vi "Parse Response.vi"(8 "error in (no error)":errorcluster, 10 "JSON Request":string, 11 "JSON-RPC in":refnum<class "JSON-RPC.lvclass">) -> (0 "error out":errorcluster, 1 "ids":string[](array[string]), 2 "Results":variant[](array[variant]), 3 "JSON-RPC out":refnum<class "JSON-RPC.lvclass">)   [LabVIEW 2016, in "JSON-RPC.lvclass"]
uses:
  JSON-RPC.lvclass
  JSON-RPC.lvclass/JSON-RPC.ctl
  Request/Request.lvclass
  <vilib>/addons/_JKI.lib/Serialization/JSON/JKI JSON Serialization.lvlib
  <vilib>/Utility/Data Type/NI_Data Type.lvlib
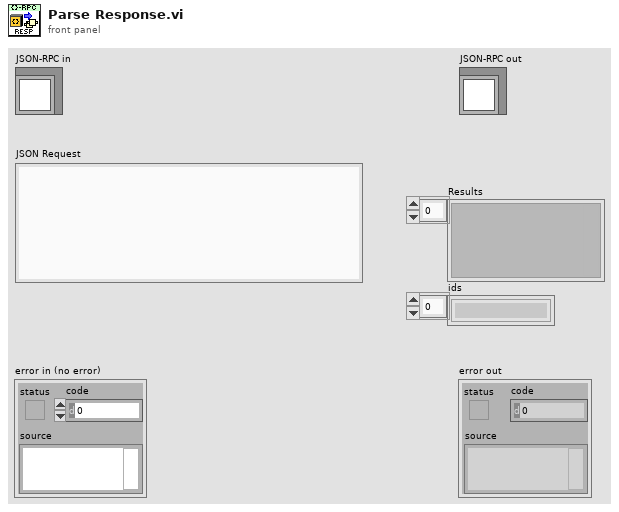
[diagram p1: front panel]
types:
  T1 = typedef "NI_Data Type.lvlib/Data Type.ctl" = enum8{"Invalid Type", "Void", "I8", "I16", "I32", "I64", "U8", "U16", "U32", "U64", "Single Float", "Double Float", "Extended Float", "Single Complex", "Double Complex", "Extended Complex", "Enum U8", "Enum U16", "Enum U32", "Enum U64", "Single Float With Unit", "Double Float With Unit", "Extended Float With Unit", "Single Complex with Unit", "Double Complex with Unit", "Extended Complex with Unit", "Boolean", "String", "Path", "Picture", "Tag", "Array", "Cluster", "Variant", "LV Variant", "Waveform", "Timestamp", "Digital Waveform", "Digital Data", "ExpressData", "Refnum", "External Data", "VI", "Poly VI", "LabVIEW Class Instance", "Fixed Point"}
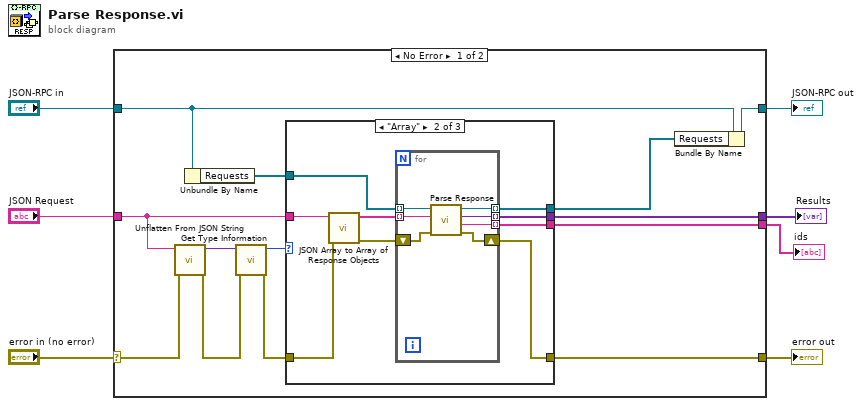
[diagram p0: block diagram]
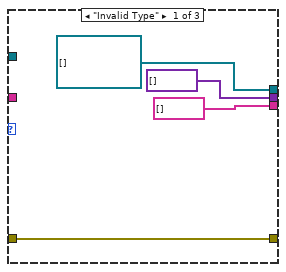
[diagram p2: hidden frame]
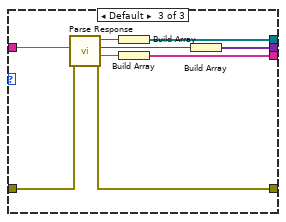
[diagram p3: hidden frame]
diagram:
  n1 = case shown="No Error" "error in (no error)" {
    selector: "error in (no error)" -> [w20 w51]
    tunnel: [w15 w51] -> w6
    tunnel: [w19 w50] -> w4
    tunnel: "JSON-RPC in" -> [w11 w50]
    tunnel: "JSON Request" -> [w13 _]
    tunnel: [w12 _] -> w2
    tunnel: [w8 _] -> w1
    frame No Error {
      n2 = call <vilib>:"Unflatten From JSON String.vi"("error in (no error)"=w20, "JSON String"=w13) -> ("error out"=w17:errorcluster, "Variant"=w16:variant)  [unwired: 8 in]
      n3 = Unbundle By Name(w11) -> ("Requests"=w10:refnum<class "Request.lvclass">[])
      n4 = call <vilib>:"Get Type Information.vi"("error in (no error)"=w17, "Variant"=w16) -> ("error out"=w14:errorcluster, "Type"=w18:T1)  [unwired: 5 in, 3 out]
      n5 = case shown="\"Array\"" w18 {
        tunnel: w14 -> [w24 w27 w48]
        tunnel: [w24 w33 w47] -> w15
        tunnel: w13 -> [_ w28 w46]
        tunnel: [variant[] [] w32 w49] -> w12
        tunnel: [refnum<class "Request.lvclass">[] [] ("Requests") w31 w43] -> w9
        tunnel: w10 -> [_ w30 _]
        tunnel: [string[] [] w29 w41] -> w8
        frame "Invalid Type" {
        }
        frame "Array" {
          n6 = call "JSON Array to Array of Response Objects.vi"("error in (no error)"=w27, "JSON Array"=w28) -> ("error out"=w26:errorcluster, "Response Objects"=w25:string[])  [unwired: 8 in]
          n7 = for {
            tunnel: [w37] -> w31 mode=indexing
            shift-right: [w39] -> w33
            shift-left: w26 -> [w40]
            tunnel: w25 -> [w36] mode=indexing
            tunnel: [w38] -> w32 mode=indexing
            tunnel: [w35] -> w29 mode=indexing
            tunnel: w30 -> [w34] mode=indexing
            n8 = call "Parse Response.vi"("error in (no error)"=w40, "JSON String"=w36, "Request"=w34) -> ("error out"=w39:errorcluster, "id"=w35:string, "result"=w38:variant, "Request out"=w37:refnum<class "Request.lvclass">)  [unwired: 5 in]
          }
        }
        frame Default {
          n9 = call "Parse Response.vi"("error in (no error)"=w48, "JSON String"=w46) -> ("error out"=w47:errorcluster, "id"=w42:string, "result"=w44:variant, "Request out"=w45:refnum<class "Request.lvclass">)  [unwired: 6 in]
          n10 = Build Array(w45) -> (w43:refnum<class "Request.lvclass">[])
          n11 = Build Array(w42) -> (w41:string[])
          n12 = Build Array(w44) -> (w49:variant[])
        }
      }
      n13 = Bundle By Name(cluster=w11, "Requests"=w9) -> (w19:refnum<class "JSON-RPC.lvclass">)
    }
    frame Error {
    }
  }
  "error out" <- w6
  "JSON-RPC out" <- w4
  "Results" <- w2
  "ids" <- w1
